vi "ChangeToDACcodes+CheckLimit.vi"(11 "Input Waveform":dbl[](array[numeric])) -> (3 "DAC Codes":u16[](array[numeric]))   [LabVIEW 2018]
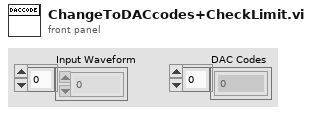
[diagram p1: front panel]
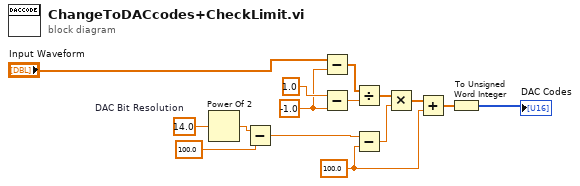
[diagram p0: block diagram]
diagram:
  w1 = -1.0 ("max value")
  w9 = 100.0 ("y")
  w13 = 14.0  # DAC Bit Resolution
  n1 = Power Of 2(x=w13) -> (2^x=w5:dbl)
  n2 = Subtract(x=w5, y=100.0) -> (x-y=w4:dbl)
  n3 = Subtract(x="Input Waveform", y=w1) -> (x-y=w15:dbl[])
  n4 = Subtract(x=1.0 ("max value"), y=w1) -> (x-y=w14:dbl)
  n5 = Divide(x=w15, y=w14) -> (x/y=w12:dbl[])
  n6 = Subtract(x=w4, y=w9) -> (x-y=w11:dbl)
  n7 = Multiply(x=w12, y=w11) -> (x*y=w10:dbl[])
  n8 = Add(x=w10, y=w9) -> (x+y=w8:dbl[])
  n9 = To Unsigned Word Integer(number=w8) -> (unsigned 16bit integer=→"DAC Codes":u16[])
